vi "Init.vi"(8 "error in (no error)":errorcluster, 11 "Snake in":refnum<class "Snake.lvclass">) -> (0 "error out":errorcluster, 3 "Snake out":refnum<class "Snake.lvclass">)   [LabVIEW 2019, in "RT_Game.lvlib" / "Snake.lvclass"]
uses:
  Snake.lvclass
  Snake.lvclass/Snake.ctl
  GameObject/GameObject.lvclass
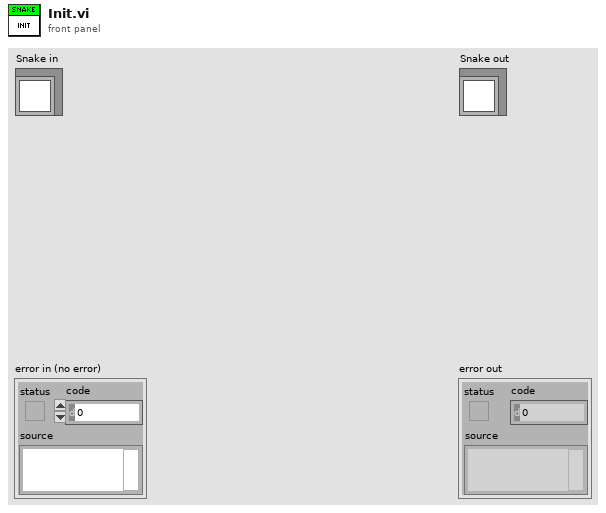
[diagram p1: front panel]
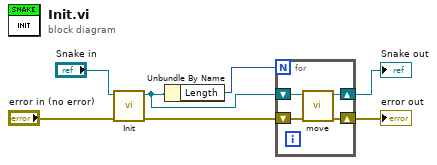
[diagram p0: block diagram]
diagram:
  n1 = call-parent "Init.vi"("error in (no error)"="error in (no error)", "GameObject in"="Snake in") -> ("error out"=w7:errorcluster, "GameObject out"=w2:refnum<class "Snake.lvclass">)  [unwired: 8 in]
  n2 = Unbundle By Name(w2) -> ("Length"=w1:i16)
  n3 = for {
    N: w1 -> [_]
    shift-right: [w10] -> w4
    shift-left: w7 -> [w11]
    shift-right: [w9] -> w3
    shift-left: w2 -> [w8]
    n4 = call "move.vi"("error in (no error)"=w11, "Snake in"=w8) -> ("error out"=w10:errorcluster, "Snake out"=w9:refnum<class "Snake.lvclass">)  [unwired: 8 in]
  }
  "error out" <- w4
  "Snake out" <- w3
